vi "Manually Configure Gyro Offset.vi"(0 "VISA resource name":refnum<visa-resource-name>, 5 "X Axis Gyro Offset (0 rad/s)":sgl, 7 "Y Axis Gyro Offset (0 rad/s)":sgl, 9 "Z Axis Gyro Offset (0 rad/s)":sgl, 11 "error in (no error)":errorcluster) -> (4 "VISA resource name out":refnum<visa-resource-name>, 15 "error out":errorcluster)   [LabVIEW 2012, in "MicroStrain 3DM-GXx.lvlib"]
doc: "The specified values of GyroOffsetX, GyroOffsetY, and GyroOffsetZ (rad/s) will be subtracted from all subsequent measurements of Angular Rate.\n\nThe above values will be stored in RAM. To save the values in non-volatile memory use the 'Transfer Calibration To EEPROM' VI after this VI."
uses:
  <instrlib>/MicroStrain 3DM-GXx/MicroStrain 3DM-GXx.lvlib
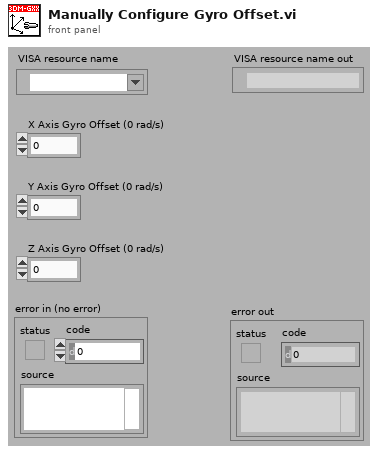
[diagram p1: front panel]
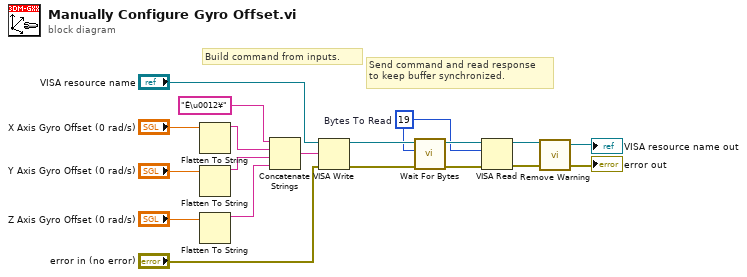
[diagram p0: block diagram]
diagram:
  w5 = u32 19  # Bytes To Read
  # "Send command and read response\nto keep buffer synchronized."
  # "Build command from inputs."
  n1 = Flatten To String(anything="X Axis Gyro Offset (0 rad/s)") -> (data string=w17:string)  [unwired: 3 in, 2 out]
  n2 = Flatten To String(anything="Y Axis Gyro Offset (0 rad/s)") -> (data string=w14:string)  [unwired: 3 in, 2 out]
  n3 = Flatten To String(anything="Z Axis Gyro Offset (0 rad/s)") -> (data string=w13:string)  [unwired: 3 in, 2 out]
  n4 = Concatenate Strings("Ê\u0012¥", w17, w14, w13) -> (w12:string)
  n5 = VISA Write(VISA resource name="VISA resource name", write buffer=w12, error in (no error)="error in (no error)") -> (VISA resource name out=w9:refnum<visa-resource-name>, error out=w8:errorcluster)  [unwired: 1 out]
  n6 = call <instrlib>:"Wait For Bytes.vi"("error in (no error)"=w8, "Bytes To Read (0)"=w5, "VISA resource name"=w9) -> ("error out"=w6:errorcluster, "VISA resource name out"=w7:refnum<visa-resource-name>)  [unwired: 7 in]
  n7 = VISA Read(VISA resource name=w7, byte count=w5, error in (no error)=w6) -> (VISA resource name out=w4:refnum<visa-resource-name>, error out=w3:errorcluster)  [unwired: 2 out]
  n8 = call <instrlib>:"Remove Warning.vi"("error in (no error)"=w3, "VISA resource name"=w4) -> ("error out"=→"error out":errorcluster, "VISA resource name out"=→"VISA resource name out":refnum<visa-resource-name>)  [unwired: 2 in]
